vi "line to strings.vi"(11 "line":T1) -> (3 "strings":string[](array[string]))   [LabVIEW 2013, in "EIP Tags editor node.lvclass"]
uses:
  EIP Tags editor node.lvclass
  table line.ctl
  <vilib>/NI/TBM Modules/EIP Tags/channel/EIP Tags Channel.lvclass
  <vilib>/NI/Tag Bus/tag/tag descriptor.lvclass/tag descriptor.ctl
  <vilib>/NI/Tag Bus Module Framework/channel/TBM channel.lvclass/TBM channel.ctl
  <vilib>/NI/TBM Modules/EIP Tags/channel/EIP Tags Channel.lvclass/EIP Tags Channel.ctl
  <vilib>/NI/TBM Modules/EIP Tags/configuration/eip tag types.ctl
  <vilib>/NI/Tag Bus/tag/read tag name.vi
  <vilib>/NI/Tag Bus Module Framework/channel/Read channel classification.vi
  <vilib>/NI/TBM Modules/EIP Tags/channel/Read EIP Tag UUID.vi
  <vilib>/NI/TBM Modules/EIP Tags/channel/Read element.vi
  <vilib>/NI/Tag Bus/tag/read data type.vi
  <vilib>/NI/TBM Modules/EIP Tags/configuration/EIP Tags Configuration.lvclass
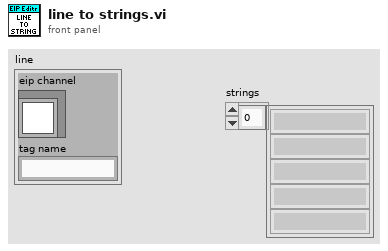
[diagram p1: front panel]
types:
  T1 = typedef "EIP Tags editor node.lvclass/table line.ctl" = cluster{"eip channel":refnum<class "EIP Tags Channel.lvclass">, "tag name":string}
  T2 = typedef "TBM channel.lvclass/channel classification.ctl" = enum16{"input data", "output data", "processing parameter", "processing result"}
  T3 = typedef "tag bus.lvlib/tag descriptor.lvclass/Data Type.ctl" = enum16{"Double", "Single", "I64", "I32", "I16", "I8", "U64", "U32", "U16", "U8", "Boolean", "String", "Array of Double", "Array of Single", "Array of I64", "Array of I32", "Array of I16", "Array of I8", "Array of U64", "Array of U32", "Array of U16", "Array of U8", "Array of Boolean", "Array of String"}
  T4 = typedef "EIP Tags Configuration.lvclass/eip tag types.ctl" = enum16{"SINT", "INT", "DINT", "REAL", "BOOL", "STRING"}
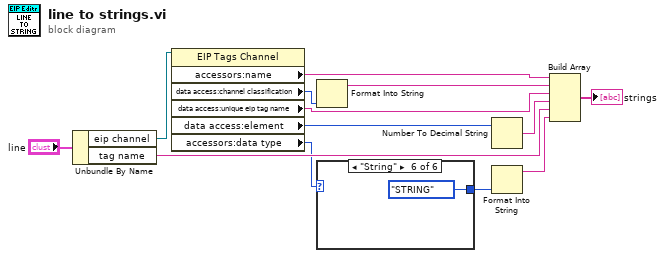
[diagram p0: block diagram]
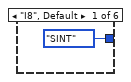
[diagram p2: hidden frame]
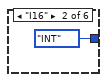
[diagram p3: hidden frame]
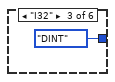
[diagram p4: hidden frame]
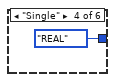
[diagram p5: hidden frame]
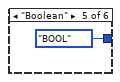
[diagram p6: hidden frame]
diagram:
  n1 = Unbundle By Name("line") -> ("eip channel"=w11:refnum<class "EIP Tags Channel.lvclass">, "tag name"=w9:string)
  n2 = property class="EIP Tags Channel"(reference=w11) -> ("accessors:name"=w10:string, "data access:channel classification"=w8:T2, "data access:unique eip tag name"=w6:string, "data access:element"=w5:i32, "accessors:data type"=w2:T3)  [unwired: 1 in, 2 out]
  n3 = Format Into String(w8) -> (resulting string=w7:string)  [unwired: 3 in, 1 out]
  n4 = case shown="\"String\"" w2 {
    tunnel: [eip_tag_types."SINT" ("eip tag type") eip_tag_types."INT" ("eip tag type") eip_tag_types."DINT" ("eip tag type") eip_tag_types."REAL" ("eip tag type") eip_tag_types."BOOL" ("eip tag type") eip_tag_types."STRING" ("eip tag type")] -> w1
    frame "I8", Default {
    }
    frame "I16" {
    }
    frame "I32" {
    }
    frame "Single" {
    }
    frame "Boolean" {
    }
    frame "String" {
    }
  }
  n5 = Number To Decimal String(number=w5) -> (decimal integer string=w4:string)  [unwired: 1 in]
  n6 = Format Into String(w1) -> (resulting string=w3:string)  [unwired: 3 in, 1 out]
  n7 = Build Array(w10, w7, w6, w4, w9, w3) -> (→"strings":string[])
